vi "ICM Read Write Format.vi"(8 "error in (no error)":errorcluster, 9 "ICM file":path, 10 "Data File":path) -> (0 "error out (no error)":errorcluster)   [LabVIEW 2024]
doc: "OSDS Read Write Format.vi\n\n This VI is used to read and write the Format header which is used in both the Format definition files and in the Streamed Data files.\n\nOCC Streaming Data System Version 1.0\nJune, 2007 Original Code Consulting David Thomson\n www.originalcode.com"
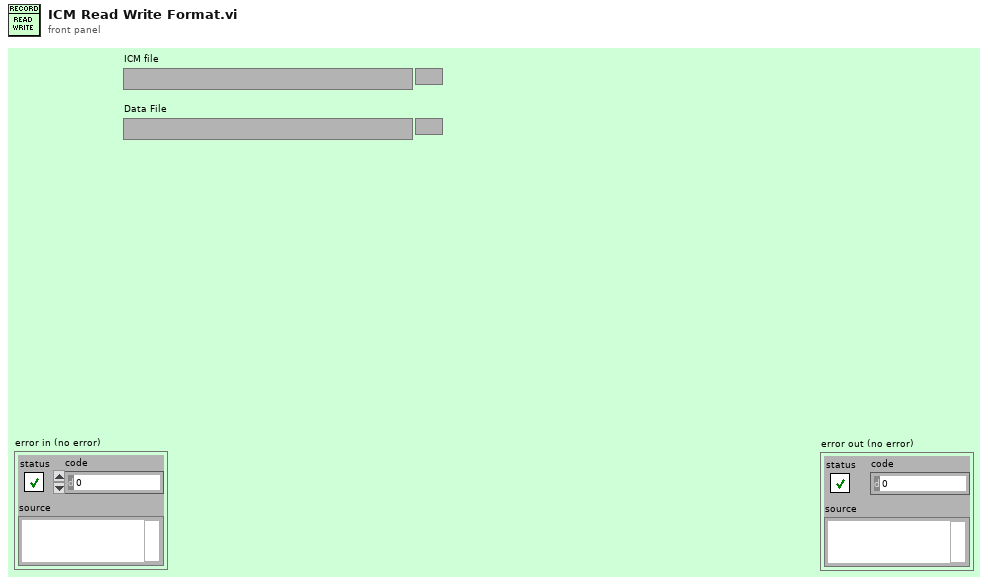
[diagram p1: front panel]
types:
  T1 = enum16{"open", "replace", "create", "open or create", "replace or create", "replace or create with confirmation"}
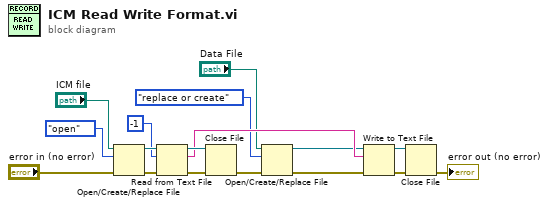
[diagram p0: block diagram]
diagram:
  n1 = Open/Create/Replace File(file path (use dialog)="ICM file", error in="error in (no error)", operation (0:open)=T1."open") -> (refnum out=w17:refnum<file>, error out=w15:errorcluster)  [unwired: 3 in, 1 out]
  n2 = Read from Text File(file (use dialog)=w17, count=-1, error in=w15) -> (refnum out=w13:refnum<file>, text=w11:string, error out=w12:errorcluster)  [unwired: 1 in, 1 out]
  n3 = Close File(refnum=w13, error in=w12) -> (error out=w5:errorcluster)  [unwired: 1 out]
  n4 = Open/Create/Replace File(file path (use dialog)="Data File", error in=w5, operation (0:open)=T1."replace or create") -> (refnum out=w9:refnum<file>, error out=w8:errorcluster)  [unwired: 3 in, 1 out]
  n5 = Write to Text File(file (use dialog)=w9, text=w11, error in=w8) -> (refnum out=w7:refnum<file>, error out=w6:errorcluster)  [unwired: 1 in, 1 out]
  n6 = Close File(refnum=w7, error in=w6) -> (error out=→"error out (no error)":errorcluster)  [unwired: 1 out]
